vi "Method.vi"(4 "Value":refnum<class "Abs_U64 Integer.lvclass">) -> (1 "Result":refnum<class "Abs_U64 Integer.lvclass">)   [LabVIEW 2021, in "Increment_U64.lvclass"]
uses:
  Increment_U64.lvclass
  Abs_Types/U64 Integer/Abs_U64 Integer.lvclass
  C:/Users/Tim/Documents/LabVIEW/2021/Data Classes/Source/Functions/Support/One Terminal/U64/AbsFunc_One Term_U64.lvclass
  C:/Users/Tim/Documents/LabVIEW/2021/Data Classes/Source/Abs_Types/U64 Integer/Abs_U64 Integer.lvclass
  Support/One Terminal/U64/AbsFunc_One Term_U64.lvclass/AbsFunc_One Term_U64.ctl
  Support/One Terminal/U64/Properties/Write Numeric A.vi
  Increment_U64.lvclass/Increment_U64.ctl
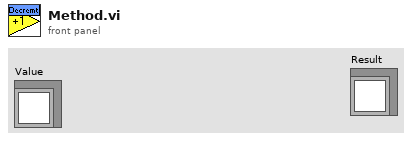
[diagram p1: front panel]
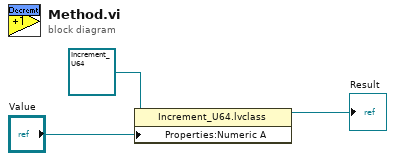
[diagram p0: block diagram]
diagram:
  n1 = property class="Increment_U64.lvclass"(reference=refnum<class "Increment_U64.lvclass"> refnum ("Decrement_DBL.lvclass"), "Properties:Numeric A"="Value") -> (reference out=→"Result":refnum<class "Increment_U64.lvclass">)  [unwired: 1 in, 1 out]
